vi "save_report_to_file.vi"() -> ()   [LabVIEW 2014]
uses:
  <vilib>/Utility/NIReport.llb/NI_report.lvclass
panel:
  in  "report file path":path
  in  "template (empty)":path
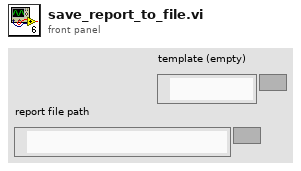
[diagram p1: front panel]
types:
  T1 = enum16{"Standard Report", "HTML", "Word", "Excel"}
  T2 = enum16{"maximized", "minimized", "normal", "no change"}
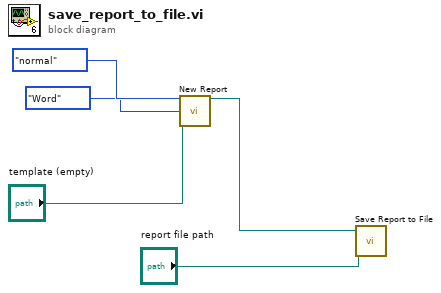
[diagram p0: block diagram]
diagram:
  n1 = call <vilib>:"New Report.vi"("window state (normal)"=T2."normal", "report type"=T1."Word", "template (empty)"="template (empty)") -> ("report out"=w2:refnum<class "NI_report.lvclass">)  [unwired: 11 in, 1 out]
  n2 = call-dynamic "Save Report to File.vi"("report in"=w2, "report file path"="report file path") -> ()  [unwired: 12 in, 2 out]
